vi "reward_behavior_michelle_visjitter_conswin_enticefx.vi"() -> ()   [LabVIEW 2019]
doc: "The myRIO Project template acquires acceleration data from the onboard accelerometer and displays the changes of acceleration values in a waveform chart."
uses:
  <vilib>/myRIO/Common/Instrument Driver Framework/Utilities/typedefs/Generic FPGA Reference.ctl
  <vilib>/myRIO/Common/Instrument Driver Framework/Utilities/typedefs/myRIO v1.0 Reference.ctl
  <vilib>/myRIO/Common/Instrument Driver Framework/Utilities/typedefs/Hardware Version Enum.ctl
  <vilib>/myRIO/Common/Instrument Driver Framework/Utilities/typedefs/myRIO Generic Hardware Reference.ctl
  <vilib>/userdefined/High Color/nirio_resource_hc.ctl
  <vilib>/myRIO/Common/Instrument Driver Framework/Utilities/vis/Is FPGA Ref Available.vi
  <vilib>/myRIO/Common/Instrument Driver Framework/myRIO v1.0/Encoder/typedefs/Encoder Signal Mode.ctl
  <vilib>/myRIO/Common/Instrument Driver Framework/myRIO v1.0/Encoder/typedefs/Encoder Channels Enum.ctl
  <vilib>/myRIO/Instrument Drivers/Onboard IO/Encoder/typedefs/Encoder Reference.ctl
  <vilib>/myRIO/Instrument Drivers/Onboard IO/Encoder/Encoder.lvlib
  <vilib>/myRIO/Instrument Drivers/Onboard IO/Encoder/vis/Read.vi
  <vilib>/myRIO/Common/Instrument Driver Framework/myRIO v1.0/Encoder/typedefs/Encoder Configuration v1.0.ctl
  <vilib>/myRIO/Common/Instrument Driver Framework/myRIO v1.0/Encoder/vis/myRIO v1.1 Open Encoder.vi
  <vilib>/myRIO/Common/Instrument Driver Framework/myRIO v1.0/Encoder/vis/myRIO v1.0 Configure Encoder.vi
  <vilib>/myRIO/Instrument Drivers/Onboard IO/Encoder/vis/myRIO Encoder Open.xnode
  <vilib>/myRIO/Express VI/Onboard IO/Encoder/Encoder Express VI.xnode
  <vilib>/myRIO/Express VI/Onboard IO/DI/DI Express VI.xnode
  <vilib>/myRIO/Instrument Drivers/Onboard IO/DIO/vis/Read.vi
  <vilib>/myRIO/Instrument Drivers/Onboard IO/DIO/DIO.lvlib
  <vilib>/myRIO/Common/Instrument Driver Framework/myRIO v1.0/DIO/typedefs/DIO Channels Enum.ctl
  <vilib>/myRIO/Common/Instrument Driver Framework/myRIO v1.0/DIO/typedefs/DIO Channels List.ctl
  <vilib>/myRIO/Instrument Drivers/Onboard IO/DIO/typedefs/DIO Reference.ctl
  <vilib>/myRIO/Instrument Drivers/Onboard IO/DIO/vis/myRIO DIO Open.xnode
  <vilib>/myRIO/Common/Instrument Driver Framework/myRIO v1.0/DIO/vis/myRIO v1.1 Open DIO.vi
  <vilib>/myRIO/Instrument Drivers/Onboard IO/DIO/vis/Write.vi
  <vilib>/myRIO/Express VI/Onboard IO/DO/DO Express VI.xnode
  <vilib>/Analysis/Matrix/Datatypes/RealMatrix.ctl
  <vilib>/Analysis/Matrix/NI_Matrix.lvlib
panel:
  out "ContrastChoice":dbl
  out "Enticements":i32
  in  "Entice":bool
  out "Misses":i32
  out "GoAhead":bool
  out "TimeOutDuration":i32
  out "ActiveTime":dbl
  out "ConsumptionGo":bool=TRUE
  out "Consumption_Period":i32
  out "Watch_Display":bool=TRUE
  in  "Give reward":bool
  out "Timings":dbl[](array[numeric])
  out "ISI":dbl
  out "ISI start time":dbl
  out "Time_out":bool=TRUE
  out "Time since lick":dbl
  out "Time of last lick":dbl
  out "Rewarded trials":dbl[](array[numeric])
  out "Rewards":u16
  out "Active Trial":bool
  out "Array temp2":T1
  out "Stimuli Loaded":bool
  out "Stim_ID":dbl[](array[numeric])
  out "Reward_mat":dbl[](array[numeric])
  out "Reward":bool=TRUE
  out "Frame clock":i32
  out "Licks":u32
  out "Lick":bool
  out "Time":dbl
  out "Stop":bool
  in  "Frames to collect":u32
  out "Overflow?":bool
  out "Counter Value":i32
  out "Velocity":dbl
  out "Velocity Plot":dbl[](graph)
  out "Velocity array":dbl[](array[numeric])
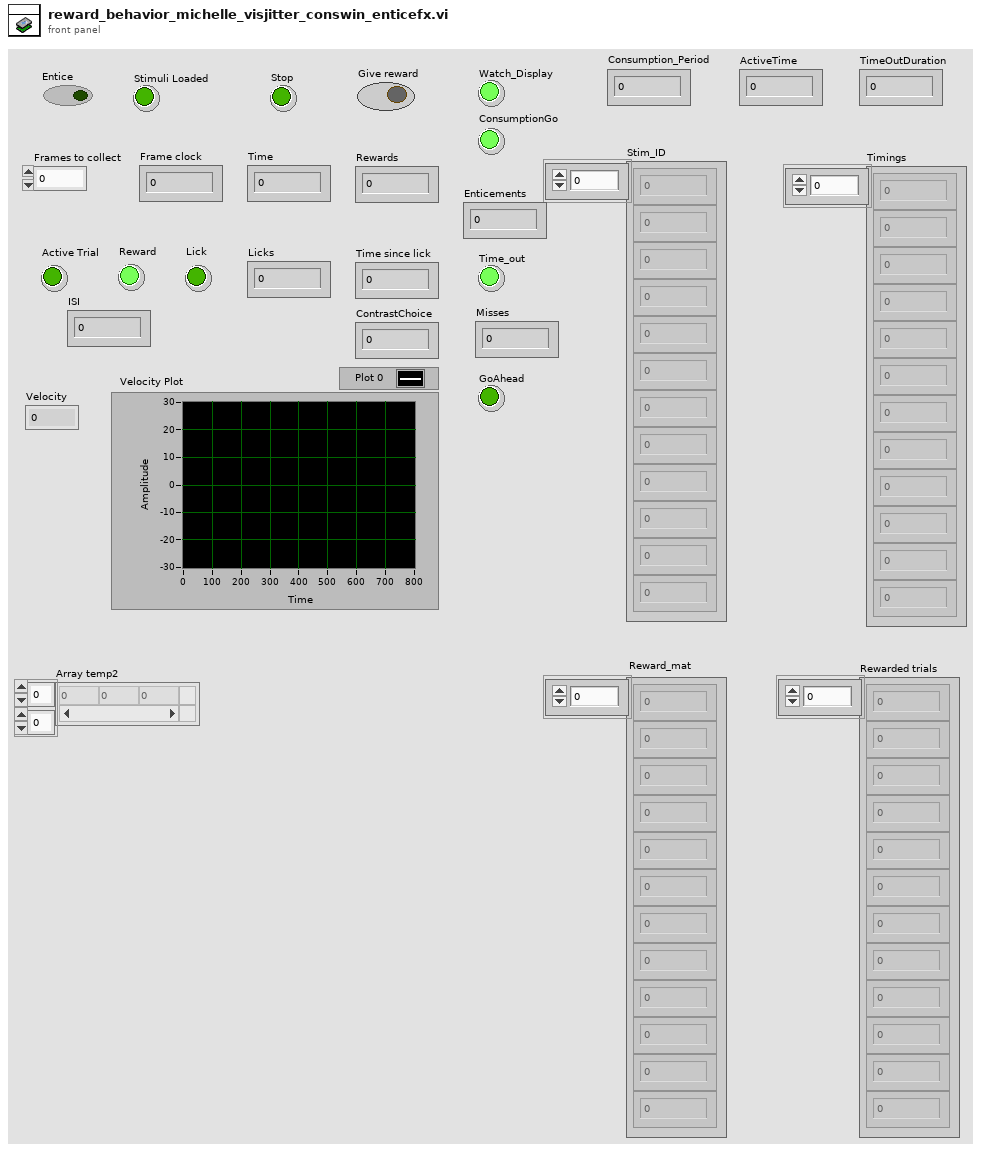
[diagram p1: front panel]
types:
  T1 = typedef "NI_Matrix.lvlib/RealMatrix.ctl" = dbl[][]
  T2 = typedef "Encoder.lvlib/Encoder Reference.ctl" = cluster{"myRIO Reference":T3, "Encoder Channels Enum":T7}
  T3 = typedef "myRIO Generic Hardware Reference.ctl" = cluster{"myRIO Model":T4, "myRIO Hardware Reference":T5}
  T4 = typedef "Hardware Version Enum.ctl" = enum16{"Unknown", "myRIO-1900", "myRIO-1950", "roboRIO", "NI ELVIS RIO CM", "ELVIS III"}
  T5 = typedef "myRIO v1.0 Reference.ctl" = cluster{"Generic FPGA Reference":T6, "Allow multiple opens":bool}
  T6 = typedef "Generic FPGA Reference.ctl" = refnum<k20>
  T7 = typedef "Encoder Channels Enum.ctl" = enum16{"Not Connected", "C/ENC0", "C/ENC1", "A/ENC", "A/ENC0", "A/ENC1", "A/ENC2", "A/ENC3", "A/ENC4", "A/ENC5", "A/ENC6", "A/ENC7", "A/ENC8", "A/ENC9", "B/ENC", "B/ENC0", "B/ENC1", "B/ENC2", "B/ENC3", "B/ENC4", "B/ENC5", "B/ENC6", "B/ENC7", "B/ENC8", "B/ENC9", "DIO/ENC0", "DIO/ENC1", "DIO/ENC2", "DIO/ENC3", "DIO/ENC4"}
  T8 = typedef "Encoder Signal Mode.ctl" = enum16{"Quadrature phase signal", "Step and direction signal"}
  T9 = typedef "nirio_resource_hc.ctl" = tag
  T10 = typedef "DIO.lvlib/DIO Reference.ctl" = cluster{"myRIO Reference":T3, "DIO Channels List":T11}
  T11 = typedef "DIO Channels List.ctl" = T12[]
  T12 = typedef "DIO Channels Enum.ctl" = enum16{"Not Connected", "C/DIO0", "C/DIO1", "C/DIO2", "C/DIO3", "C/DIO4", "C/DIO5", "C/DIO6", "C/DIO7", "A/DIO0", "A/DIO1", "A/DIO2", "A/DIO3", "A/DIO4", "A/DIO5", "A/DIO6", "A/DIO7", "A/DIO8", "A/DIO9", "A/DIO10", "A/DIO11", "A/DIO12", "A/DIO13", "A/DIO14", "A/DIO15", "A/DIO16", "A/DIO17", "A/DIO18", "A/DIO19", "B/DIO0", "B/DIO1", "B/DIO2", "B/DIO3", "B/DIO4", "B/DIO5", "B/DIO6", "B/DIO7", "B/DIO8", "B/DIO9", "B/DIO10", "B/DIO11", "B/DIO12", "B/DIO13", "B/DIO14", "B/DIO15", "B/DIO16", "B/DIO17", "B/DIO18", "B/DIO19", "LED0", "LED1", "LED2", "LED3", "Button0", "DIO/DIO0", "DIO/DIO1", "DIO/DIO2", "DIO/DIO3", "DIO/DIO4", "DIO/DIO5", "DIO/DIO6", "DIO/DIO7", "DIO/DIO8", "DIO/DIO9", "SPI/CS0", "SPI/CS1", "SPI/CS2", "SPI/CS3", "LED RADIO (Green)", "LED RADIO (Red)", "LED COMM (Green)", "LED COMM (Red)", "LED MODE (Green)", "LED MODE (Red)"}
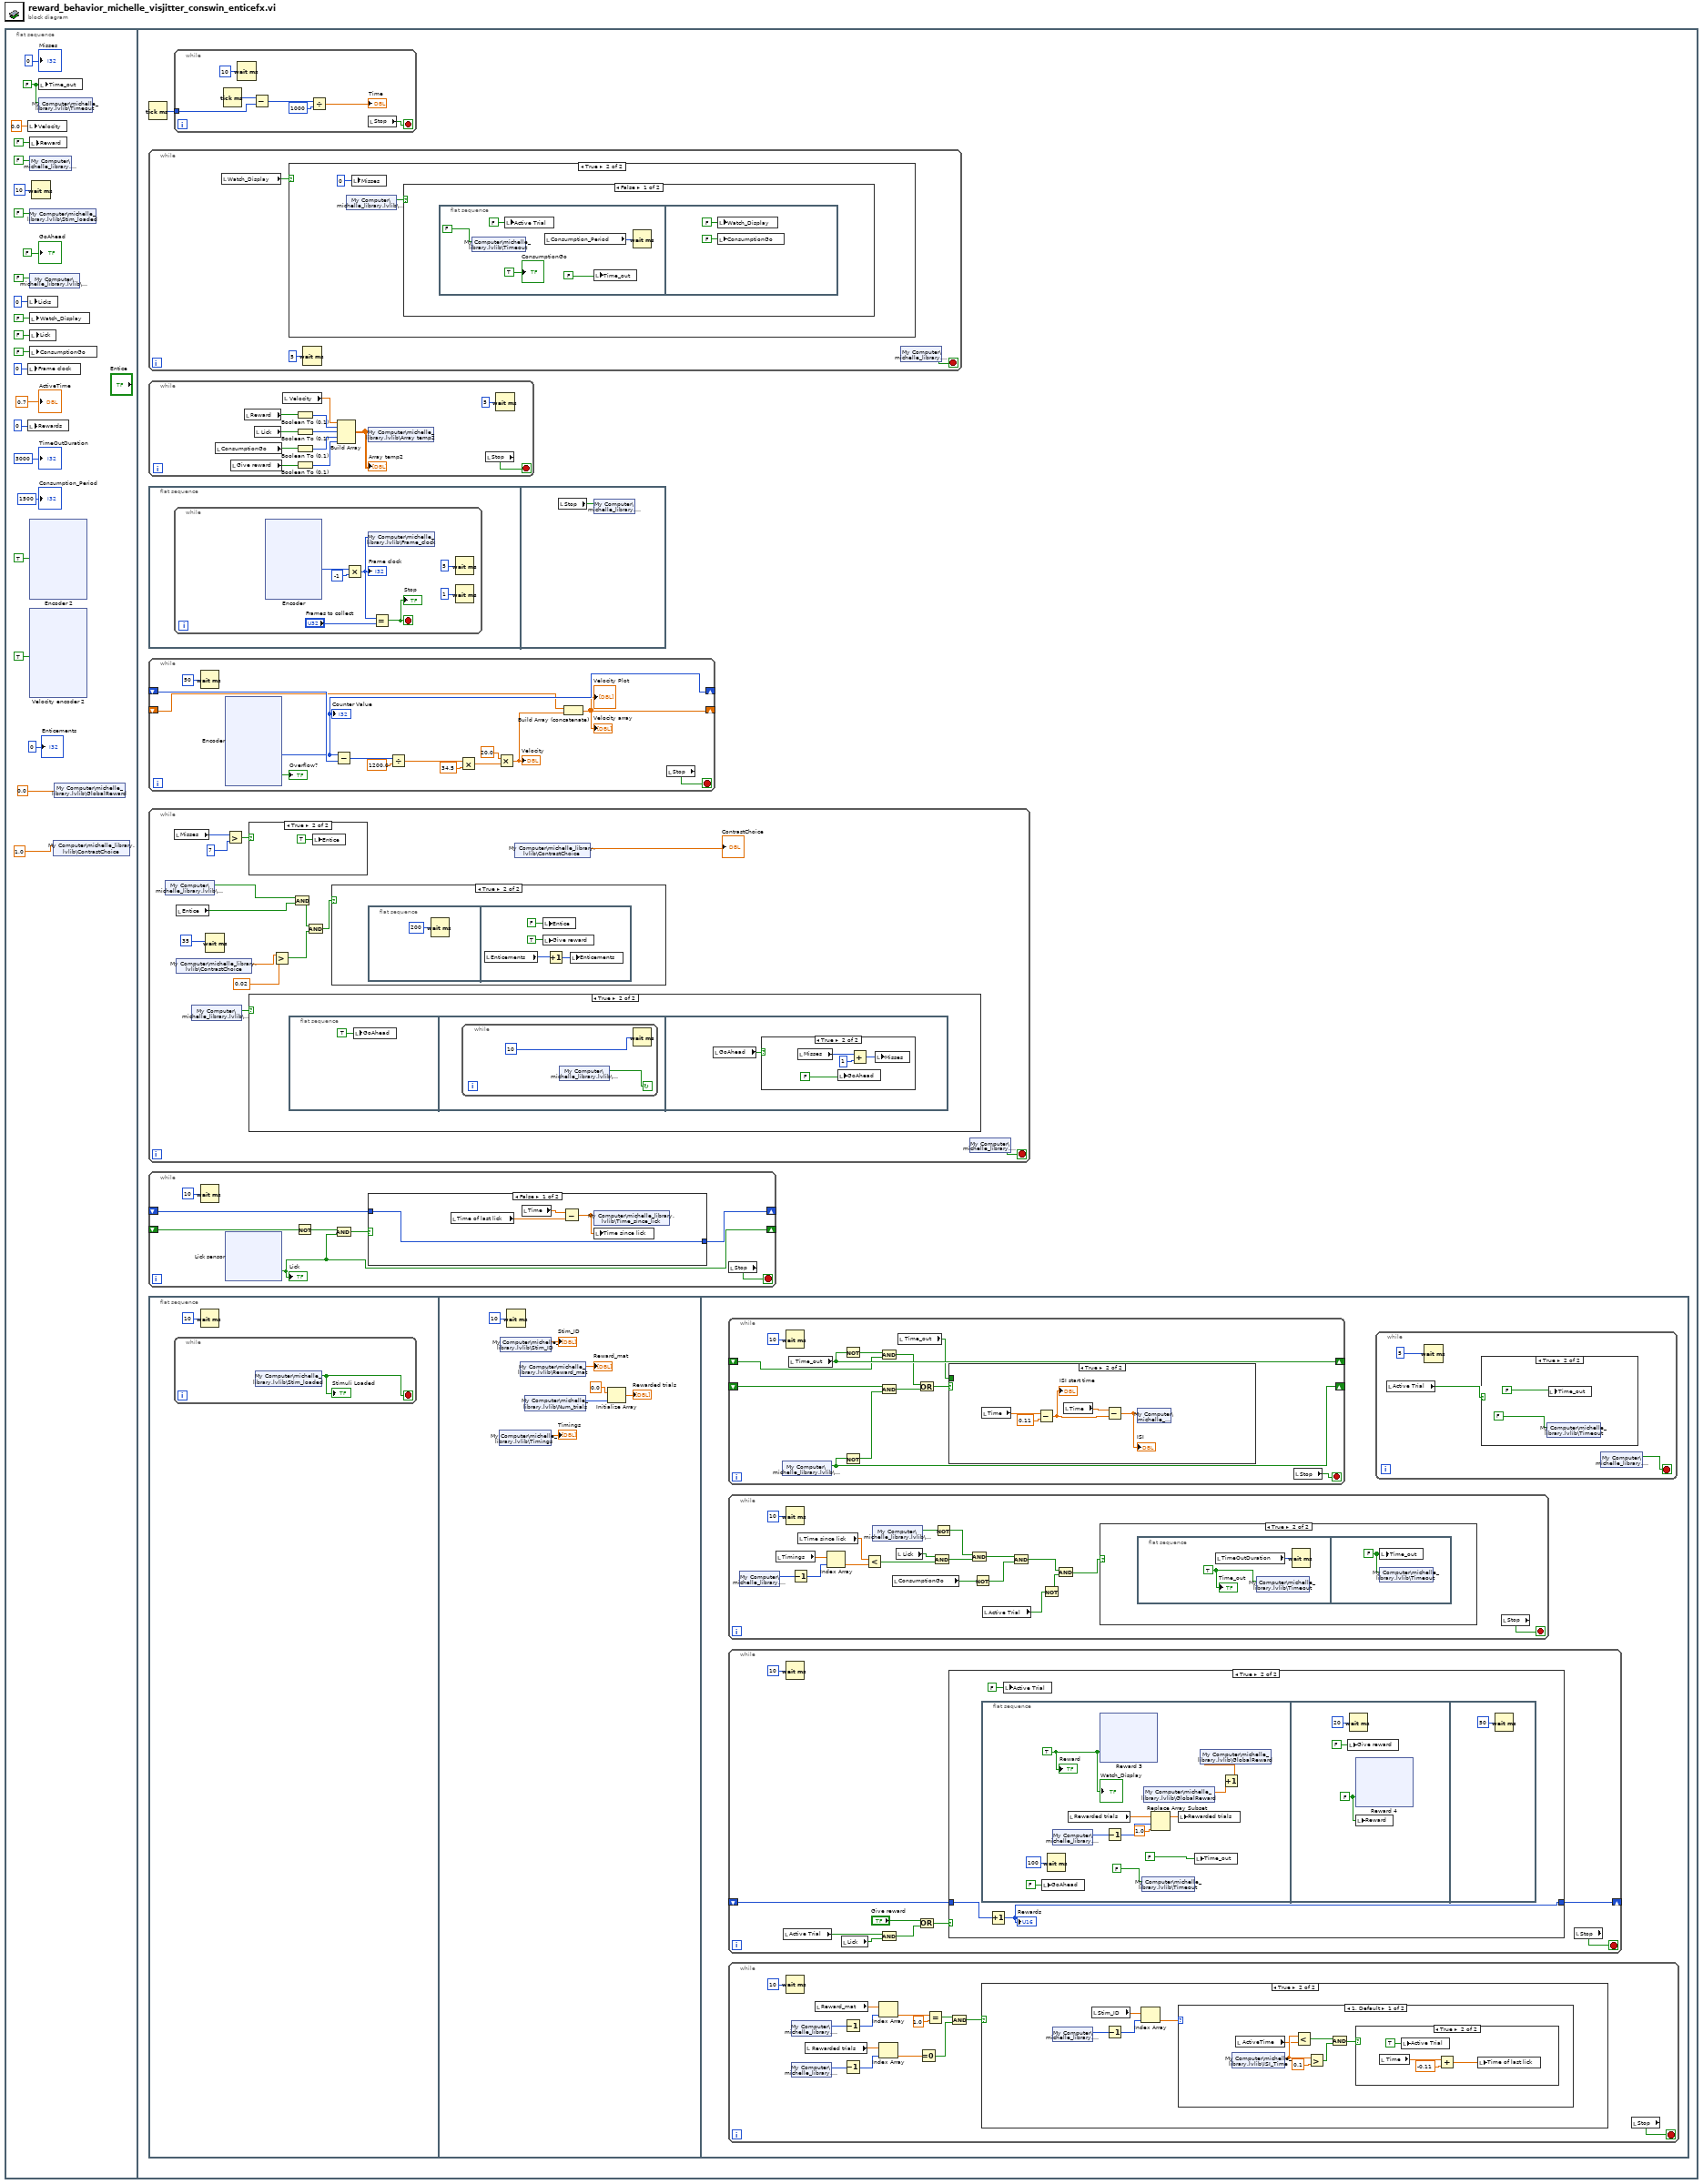
[diagram p0: block diagram]
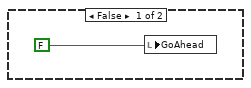
[diagram p4: hidden frame]
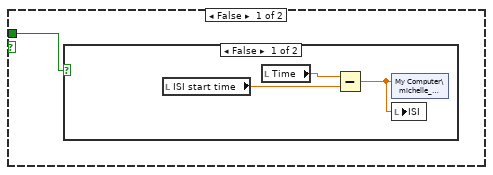
[diagram p10: hidden frame]
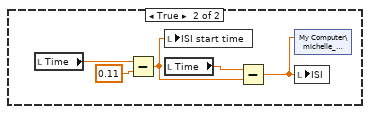
[diagram p11: hidden frame]
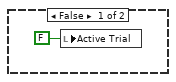
[diagram p12: hidden frame]
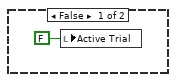
[diagram p13: hidden frame]
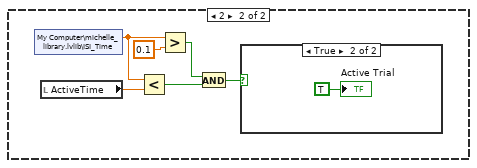
[diagram p14: hidden frame]
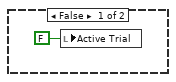
[diagram p15: hidden frame]
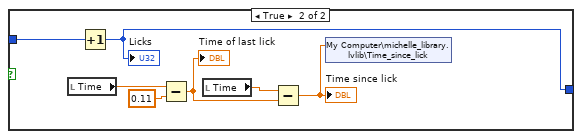
[diagram p17: hidden frame]
diagram:
  n1 = flat-sequence {
    frame #0 {
      w11 = FALSE ("Time_out")
      n2 = local write "Velocity"(0.0 ("Velocity")) -> ()
      n3 = local write "Licks"(u32 0 ("Licks")) -> ()
      n4 = local write "Frame clock"(u32 0 ("Frames")) -> ()
      n5 = local write "Rewards"(u16 0 ("Rewards")) -> ()
      n6 = local write "Reward"(FALSE ("Give reward")) -> ()
      n7 = shared-variable "My Computer\\michelle_library.lvlib\\Stop"(FALSE ("Stop")) -> ()  [unwired: 1 in, 1 out]
      n8 = shared-variable "My Computer\\michelle_library.lvlib\\Stim_loaded"(FALSE ("Stim_loaded")) -> ()  [unwired: 1 in, 1 out]
      n9 = shared-variable "My Computer\\michelle_library.lvlib\\Display"(FALSE ("Display")) -> ()  [unwired: 1 in, 1 out]
      n10 = local write "Watch_Display"(FALSE ("Watch_Display")) -> ()
      n11 = local write "Lick"(FALSE ("Lick")) -> ()
      n12 = local write "ConsumptionGo"(FALSE ("ConsumptionGo")) -> ()
      n13 = xnode "Encoder 2"("Reset Counter"=TRUE) -> ()  [unwired: 1 in, 4 out]
      n14 = xnode "Velocity encoder 2"("Reset Counter"=TRUE) -> ()  [unwired: 1 in, 4 out]
      n15 = Wait (ms)(milliseconds to wait=u32 10) -> ()  [unwired: 1 out]
      n16 = local write "Time_out"(w11) -> ()
      n17 = shared-variable "My Computer\\michelle_library.lvlib\\Timeout"(w11) -> ()  [unwired: 1 in, 1 out]
      n18 = shared-variable "My Computer\\michelle_library.lvlib\\ContrastChoice"(1.0) -> ()  [unwired: 1 in, 1 out]
      n19 = shared-variable "My Computer\\michelle_library.lvlib\\GlobalReward"(0.0) -> ()  [unwired: 1 in, 1 out]
      "Consumption_Period" <- 1500
      "ActiveTime" <- 0.7
      "TimeOutDuration" <- 3000
      "GoAhead" <- FALSE
      "Misses" <- 0
      "Enticements" <- 0
    }
    frame #1 {
      n20 = Tick Count (ms)() -> (millisecond timer value=w116:u32)
      n21 = while {
        stop <- w148 stop-if-true
        n22 = local read "Watch_Display"() -> (w147:bool)
        n23 = case shown="True" w147 {
          frame False {
          }
          frame True {
            n24 = shared-variable "My Computer\\michelle_library.lvlib\\Display"() -> (w150:bool)  [unwired: 1 in, 1 out]
            n25 = local write "Misses"(0) -> ()
            n26 = case shown="False" w150 {
              frame False {
                n27 = flat-sequence {
                  frame #0 {
                    n28 = shared-variable "My Computer\\michelle_library.lvlib\\Timeout"(FALSE) -> ()  [unwired: 1 in, 1 out]
                    n29 = local write "Active Trial"(FALSE) -> ()
                    n30 = local read "Consumption_Period"() -> (w155:i32)
                    n31 = local write "Time_out"(FALSE) -> ()
                    n32 = Wait (ms)(milliseconds to wait=w155) -> ()  [unwired: 1 out]
                    "ConsumptionGo" <- TRUE
                  }
                  frame #1 {
                    n33 = local write "Watch_Display"(FALSE ("Watch_Display")) -> ()
                    n34 = local write "ConsumptionGo"(FALSE ("ConsumptionGo")) -> ()
                  }
                }
              }
              frame True {
              }
            }
          }
        }
        n35 = Wait (ms)(milliseconds to wait=u32 5) -> ()  [unwired: 1 out]
        n36 = shared-variable "My Computer\\michelle_library.lvlib\\Stop"() -> (w148:bool)  [unwired: 1 in, 1 out]
      }
      n37 = while {
        stop <- w163 stop-if-true
        n38 = local read "ConsumptionGo"() -> (w161:bool)
        n39 = local read "Give reward"() -> (w160:bool)
        n40 = local read "Reward"() -> (w168:bool)
        n41 = local read "Lick"() -> (w169:bool)
        n42 = local read "Velocity"() -> (w167:dbl)
        n43 = Boolean To (0,1)(Boolean=w168) -> (0, 1=w166:i16)
        n44 = Boolean To (0,1)(Boolean=w169) -> (0, 1=w165:i16)
        n45 = Boolean To (0,1)(Boolean=w161) -> (0, 1=w159:i16)
        n46 = Boolean To (0,1)(Boolean=w160) -> (0, 1=w158:i16)
        n47 = Build Array(w167, w166, w165, w159, w158) -> (w162:T1)
        "Array temp2" <- w162
        n48 = shared-variable "My Computer\\michelle_library.lvlib\\Array temp2"(w162) -> ()  [unwired: 1 in, 1 out]
        n49 = local read "Stop"() -> (w163:bool)
        n50 = Wait (ms)(milliseconds to wait=u32 5) -> ()  [unwired: 1 out]
      }
      n51 = flat-sequence {
        frame #0 {
          n52 = while {
            stop <- w370 stop-if-true
            n53 = xnode "Encoder"() -> ("Counter Value"=w374:i32)  [unwired: 2 in, 3 out]
            n54 = Multiply(x=w374, y=-1) -> (x*y=w369:i32)
            "Frame clock" <- w369
            n55 = shared-variable "My Computer\\michelle_library.lvlib\\Frame_clock"(w369) -> ()  [unwired: 1 in, 1 out]
            n56 = Equal?(x=w369, y="Frames to collect") -> (x = y?=w370:bool)
            "Stop" <- w370
            n57 = Wait (ms)(milliseconds to wait=u32 5) -> ()  [unwired: 1 out]
            n58 = Wait (ms)(milliseconds to wait=u32 1) -> ()  [unwired: 1 out]
          }
        }
        frame #1 {
          n59 = local read "Stop"() -> (w422:bool)
          n60 = shared-variable "My Computer\\michelle_library.lvlib\\Stop"(w422) -> ()  [unwired: 1 in, 1 out]
        }
      }
      n61 = while {
        shift-right: [w487] -> _
        shift-left: _ -> [w488]
        shift-right: [w479] -> _
        shift-left: _ -> [w478]
        stop <- w477 stop-if-true
        n62 = Wait (ms)(milliseconds to wait=u32 50) -> ()  [unwired: 1 out]
        n63 = xnode "Encoder"() -> ("Counter Value"=w487:i32, "Overflow?"=→"Overflow?":bool)  [unwired: 2 in, 2 out]
        "Counter Value" <- w487
        n64 = Subtract(x=w487, y=w488) -> (x-y=w480:i32)
        n65 = Divide(x=w480, y=1200.0 ("600")) -> (x/y=w485:dbl)
        n66 = Multiply(x=w485, y=34.5) -> (x*y=w483:dbl)
        n67 = Multiply(x=20.0, y=w483) -> (x*y=w481:dbl)
        "Velocity" <- w481
        n68 = Build Array (concatenate)(w478, w481) -> (w479:dbl[])
        "Velocity Plot" <- w479
        "Velocity array" <- w479
        n69 = local read "Stop"() -> (w477:bool)
      }
      n70 = while {
        stop <- w130 stop-if-true
        n71 = shared-variable "My Computer\\michelle_library.lvlib\\Display"() -> (w125:bool)  [unwired: 1 in, 1 out]
        n72 = local read "Misses"() -> (w128:i32)
        n73 = shared-variable "My Computer\\michelle_library.lvlib\\ContrastChoice"() -> (w122:dbl)  [unwired: 1 in, 1 out]
        n74 = local read "Entice"() -> (w124:bool)
        n75 = shared-variable "My Computer\\michelle_library.lvlib\\Display"() -> (w129:bool)  [unwired: 1 in, 1 out]
        n76 = Wait (ms)(milliseconds to wait=35) -> ()  [unwired: 1 out]
        n77 = Greater?(x=w128, y=7) -> (0:w126:bool)
        n78 = case shown="True" w126 {
          frame False {
          }
          frame True {
            n79 = local write "Entice"(TRUE) -> ()
          }
        }
        n80 = case shown="True" w129 {
          frame False {
            n81 = local write "GoAhead"(FALSE) -> ()
          }
          frame True {
            n82 = flat-sequence {
              frame #0 {
                n83 = local write "GoAhead"(TRUE) -> ()
              }
              frame #1 {
                n84 = while {
                  stop <- w140 continue-if-true
                  n85 = shared-variable "My Computer\\michelle_library.lvlib\\Display"() -> (w140:bool)  [unwired: 1 in, 1 out]
                  n86 = Wait (ms)(milliseconds to wait=10) -> ()  [unwired: 1 out]
                }
              }
              frame #2 {
                n87 = local read "GoAhead"() -> (w141:bool)
                n88 = case shown="True" w141 {
                  frame False {
                  }
                  frame True {
                    n89 = local read "Misses"() -> (w145:i32)
                    n90 = local write "GoAhead"(FALSE) -> ()
                    n91 = Add(x=w145, y=1) -> (x+y=w143:i32)
                    n92 = local write "Misses"(w143) -> ()
                  }
                }
              }
            }
          }
        }
        n93 = Greater?(x=w122, y=0.02) -> (0:w119:bool)
        n94 = And(x=w125, y=w124) -> (x .and. y?=w120:bool)
        n95 = And(x=w120, y=w119) -> (x .and. y?=w118:bool)
        n96 = case shown="True" w118 {
          frame False {
          }
          frame True {
            n97 = flat-sequence {
              frame #0 {
                n98 = Wait (ms)(milliseconds to wait=200) -> ()  [unwired: 1 out]
              }
              frame #1 {
                n99 = local read "Enticements"() -> (w133:i32)
                n100 = local write "Entice"(FALSE) -> ()
                n101 = local write "Give reward"(TRUE) -> ()
                n102 = Increment(x=w133) -> (x+1=w132:i32)
                n103 = local write "Enticements"(w132) -> ()
              }
            }
          }
        }
        n104 = shared-variable "My Computer\\michelle_library.lvlib\\ContrastChoice"() -> (→"ContrastChoice":dbl)  [unwired: 1 in, 1 out]
        n105 = shared-variable "My Computer\\michelle_library.lvlib\\Stop"() -> (w130:bool)  [unwired: 1 in, 1 out]
      }
      n106 = while {
        shift-right: [w429] -> _
        shift-left: _ -> [w428]
        shift-right: [w423] -> _
        shift-left: _ -> [w426]
        stop <- w427 stop-if-true
        n107 = Wait (ms)(milliseconds to wait=u32 10) -> ()  [unwired: 1 out]
        n108 = xnode "Lick sensor"() -> ("C/DIO1 (DIO1)"=w423:bool)  [unwired: 1 in, 1 out]
        "Lick" <- w423
        n109 = Not(x=w426) -> (.not. x?=w425:bool)
        n110 = And(x=w425, y=w423) -> (x .and. y?=w424:bool)
        n111 = case shown="False" w424 {
          tunnel: [w434 w441] -> w429
          tunnel: w428 -> [w434 w440]
          frame False {
            n112 = local read "Time of last lick"() -> (w432:dbl)
            n113 = local read "Time"() -> (w433:dbl)
            n114 = Subtract(x=w433, y=w432) -> (x-y=w431:dbl)
            n115 = shared-variable "My Computer\\michelle_library.lvlib\\Time_since_lick"(w431) -> ()  [unwired: 1 in, 1 out]
            n116 = local write "Time since lick"(w431) -> ()
          }
          frame True {
            n117 = local read "Time"() -> (w437:dbl)
            n118 = Increment(x=w440) -> (x+1=w441:u32)
            "Licks" <- w441
            n119 = Subtract(x=w437, y=0.11) -> (x-y=w435:dbl)
            "Time of last lick" <- w435
            n120 = local read "Time"() -> (w439:dbl)
            n121 = Subtract(x=w439, y=w435) -> (x-y=w438:dbl)
            "Time since lick" <- w438
            n122 = shared-variable "My Computer\\michelle_library.lvlib\\Time_since_lick"(w438) -> ()  [unwired: 1 in, 1 out]
          }
        }
        n123 = local read "Stop"() -> (w427:bool)
      }
      n124 = flat-sequence {
        frame #0 {
          n125 = while {
            stop <- w171 stop-if-true
            n126 = shared-variable "My Computer\\michelle_library.lvlib\\Stim_loaded"() -> (w171:bool)  [unwired: 1 in, 1 out]
            "Stimuli Loaded" <- w171
          }
          n127 = Wait (ms)(milliseconds to wait=u32 10) -> ()  [unwired: 1 out]
        }
        frame #1 {
          n128 = shared-variable "My Computer\\michelle_library.lvlib\\Timings"() -> (→"Timings":dbl[])  [unwired: 1 in, 1 out]
          n129 = shared-variable "My Computer\\michelle_library.lvlib\\Stim_ID"() -> (→"Stim_ID":dbl[])  [unwired: 1 in, 1 out]
          n130 = Wait (ms)(milliseconds to wait=u32 10) -> ()  [unwired: 1 out]
          n131 = shared-variable "My Computer\\michelle_library.lvlib\\Reward_mat"() -> (→"Reward_mat":dbl[])  [unwired: 1 in, 1 out]
          n132 = shared-variable "My Computer\\michelle_library.lvlib\\Num_trials"() -> (w175:u32)  [unwired: 1 in, 1 out]
          n133 = Initialize Array(0.0 ("element"), w175) -> (→"Rewarded trials":dbl[])
        }
        frame #2 {
          n134 = while {
            shift-right: [w216] -> _
            shift-left: _ -> [w214]
            shift-right: [w212] -> _
            shift-left: _ -> [w211]
            stop <- w217 stop-if-true
            n135 = shared-variable "My Computer\\michelle_library.lvlib\\Display"() -> (w212:bool)  [unwired: 1 in, 1 out]
            n136 = Wait (ms)(milliseconds to wait=u32 10) -> ()  [unwired: 1 out]
            n137 = local read "Time_out"() -> (w216:bool)
            n138 = Not(x=w216) -> (.not. x?=w215:bool)
            n139 = Not(x=w212) -> (.not. x?=w210:bool)
            n140 = And(x=w215, y=w214) -> (x .and. y?=w209:bool)
            n141 = And(x=w211, y=w210) -> (x .and. y?=w208:bool)
            n142 = local read "Time_out"() -> (w213:bool)
            n143 = Or(x=w209, y=w208) -> (x .or. y?=w207:bool)
            n144 = case shown="True" w207 {
              tunnel: w213 -> [w218 _]
              frame False {
                n145 = case shown="False" w218 {
                  frame False {
                    n146 = local read "ISI start time"() -> (w221:dbl)
                    n147 = local read "Time"() -> (w220:dbl)
                    n148 = Subtract(x=w220, y=w221) -> (x-y=w219:dbl)
                    n149 = shared-variable "My Computer\\michelle_library.lvlib\\ISI"(w219) -> ()  [unwired: 1 in, 1 out]
                    n150 = local write "ISI"(w219) -> ()
                  }
                  frame True {
                    n151 = local read "Time"() -> (w226:dbl)
                    n152 = Subtract(x=w226, y=0.11) -> (x-y=w223:dbl)
                    n153 = local write "ISI start time"(w223) -> ()
                    n154 = local read "Time"() -> (w224:dbl)
                    n155 = Subtract(x=w224, y=w223) -> (x-y=w222:dbl)
                    n156 = shared-variable "My Computer\\michelle_library.lvlib\\ISI"(w222) -> ()  [unwired: 1 in, 1 out]
                    n157 = local write "ISI"(w222) -> ()
                  }
                }
              }
              frame True {
                n158 = local read "Time"() -> (w231:dbl)
                n159 = Subtract(x=w231, y=0.11) -> (x-y=w228:dbl)
                "ISI start time" <- w228
                n160 = local read "Time"() -> (w229:dbl)
                n161 = Subtract(x=w229, y=w228) -> (x-y=w227:dbl)
                "ISI" <- w227
                n162 = shared-variable "My Computer\\michelle_library.lvlib\\ISI"(w227) -> ()  [unwired: 1 in, 1 out]
              }
            }
            n163 = local read "Stop"() -> (w217:bool)
          }
          n164 = while {
            stop <- w202 stop-if-true
            n165 = shared-variable "My Computer\\michelle_library.lvlib\\Trial"() -> (w192:u32)  [unwired: 1 in, 1 out]
            n166 = local read "Timings"() -> (w194:dbl[])
            n167 = Wait (ms)(milliseconds to wait=u32 10) -> ()  [unwired: 1 out]
            n168 = Decrement(x=w192) -> (x-1=w191:u32)
            n169 = local read "Time since lick"() -> (w201:dbl)
            n170 = Index Array(array=w194, index=w191) -> (element=w193:dbl)
            n171 = Less?(x=w201, y=w193) -> (x < y?=w200:bool)
            n172 = shared-variable "My Computer\\michelle_library.lvlib\\Display"() -> (w197:bool)  [unwired: 1 in, 1 out]
            n173 = local read "ConsumptionGo"() -> (w189:bool)
            n174 = local read "Lick"() -> (w199:bool)
            n175 = And(x=w199, y=w200) -> (x .and. y?=w195:bool)
            n176 = Not(x=w197) -> (.not. x?=w196:bool)
            n177 = And(x=w196, y=w195) -> (x .and. y?=w188:bool)
            n178 = Not(x=w189) -> (.not. x?=w190:bool)
            n179 = local read "Active Trial"() -> (w184:bool)
            n180 = And(x=w188, y=w190) -> (x .and. y?=w186:bool)
            n181 = Not(x=w184) -> (.not. x?=w187:bool)
            n182 = And(x=w186, y=w187) -> (x .and. y?=w185:bool)
            n183 = case shown="True" w185 {
              frame False {
              }
              frame True {
                n184 = flat-sequence {
                  frame #0 {
                    w204 = TRUE
                    n185 = local read "TimeOutDuration"() -> (w203:i32)
                    n186 = shared-variable "My Computer\\michelle_library.lvlib\\Timeout"(w204) -> ()  [unwired: 1 in, 1 out]
                    n187 = Wait (ms)(milliseconds to wait=w203) -> ()  [unwired: 1 out]
                    "Time_out" <- w204
                  }
                  frame #1 {
                    w205 = FALSE ("Timeout")
                    n188 = local write "Time_out"(w205) -> ()
                    n189 = shared-variable "My Computer\\michelle_library.lvlib\\Timeout"(w205) -> ()  [unwired: 1 in, 1 out]
                  }
                }
              }
            }
            n190 = local read "Stop"() -> (w202:bool)
          }
          n191 = while {
            shift-right: [w276] -> _
            shift-left: _ -> [w275]
            stop <- w278 stop-if-true
            n192 = local read "Active Trial"() -> (w273:bool)
            n193 = Wait (ms)(milliseconds to wait=u32 10) -> ()  [unwired: 1 out]
            n194 = local read "Lick"() -> (w274:bool)
            n195 = And(x=w273, y=w274) -> (x .and. y?=w272:bool)
            n196 = Or(x="Give reward", y=w272) -> (x .or. y?=w271:bool)
            n197 = case shown="True" w271 {
              tunnel: [w279 w282] -> w276
              tunnel: w275 -> [w279 w281]
              frame False {
              }
              frame True {
                n198 = flat-sequence {
                  frame #0 {
                    w293 = TRUE ("C/DIO0 (DIO0)")
                    n199 = local write "GoAhead"(FALSE) -> ()
                    n200 = Wait (ms)(milliseconds to wait=u32 100) -> ()  [unwired: 1 out]
                    n201 = shared-variable "My Computer\\michelle_library.lvlib\\Trial"() -> (w292:u32)  [unwired: 1 in, 1 out]
                    n202 = local read "Rewarded trials"() -> (w290:dbl[])
                    n203 = xnode "Reward 3"("C/DIO0 (DIO0)"=w293) -> ()  [unwired: 1 in, 1 out]
                    n204 = Decrement(x=w292) -> (x-1=w291:u32)
                    n205 = shared-variable "My Computer\\michelle_library.lvlib\\Timeout"(FALSE) -> ()  [unwired: 1 in, 1 out]
                    n206 = shared-variable "My Computer\\michelle_library.lvlib\\GlobalReward"() -> (w284:dbl)  [unwired: 1 in, 1 out]
                    n207 = Replace Array Subset(array=w290, new element=1.0 ("new element/subarray"), index=w291) -> (w288:dbl[])
                    n208 = local write "Rewarded trials"(w288) -> ()
                    n209 = local write "Time_out"(FALSE) -> ()
                    n210 = Increment(x=w284) -> (x+1=w283:dbl)
                    n211 = shared-variable "My Computer\\michelle_library.lvlib\\GlobalReward"(w283) -> ()  [unwired: 1 in, 1 out]
                    "Reward" <- w293
                    "Watch_Display" <- w293
                  }
                  frame #1 {
                    w332 = FALSE ("C/DIO0 (DIO0)")
                    n212 = local write "Give reward"(FALSE ("Give reward")) -> ()
                    n213 = Wait (ms)(milliseconds to wait=u32 20) -> ()  [unwired: 1 out]
                    n214 = xnode "Reward 4"("C/DIO0 (DIO0)"=w332) -> ()  [unwired: 1 in, 1 out]
                    n215 = local write "Reward"(w332) -> ()
                  }
                  frame #2 {
                    n216 = Wait (ms)(milliseconds to wait=u32 50) -> ()  [unwired: 1 out]
                  }
                }
                n217 = Increment(x=w281) -> (x+1=w282:u16)
                "Rewards" <- w282
                n218 = local write "Active Trial"(FALSE ("Active Trial")) -> ()
              }
            }
            n219 = local read "Stop"() -> (w278:bool)
          }
          n220 = while {
            stop <- w245 stop-if-true
            n221 = Wait (ms)(milliseconds to wait=u32 10) -> ()  [unwired: 1 out]
            n222 = shared-variable "My Computer\\michelle_library.lvlib\\Trial"() -> (w241:u32)  [unwired: 1 in, 1 out]
            n223 = shared-variable "My Computer\\michelle_library.lvlib\\Trial"() -> (w237:u32)  [unwired: 1 in, 1 out]
            n224 = local read "Rewarded trials"() -> (w238:dbl[])
            n225 = local read "Reward_mat"() -> (w240:dbl[])
            n226 = Decrement(x=w241) -> (x-1=w242:u32)
            n227 = Decrement(x=w237) -> (x-1=w236:u32)
            n228 = Index Array(array=w240, index=w242) -> (element=w243:dbl)
            n229 = Index Array(array=w238, index=w236) -> (element=w235:dbl)
            n230 = Equal To 0?(x=w235) -> (x = 0?=w234:bool)
            n231 = Equal?(x=w243, y=1.0) -> (x = y?=w233:bool)
            n232 = And(x=w233, y=w234) -> (x .and. y?=w232:bool)
            n233 = case shown="True" w232 {
              frame False {
                n234 = local write "Active Trial"(FALSE ("Active_trial")) -> ()
              }
              frame True {
                n235 = shared-variable "My Computer\\michelle_library.lvlib\\Trial"() -> (w248:u32)  [unwired: 1 in, 1 out]
                n236 = local read "Stim_ID"() -> (w250:dbl[])
                n237 = Decrement(x=w248) -> (x-1=w249:u32)
                n238 = Index Array(array=w250, index=w249) -> (element=w247:dbl)
                n239 = case shown="1, Default" w247 {
                  frame 1, Default {
                    n240 = shared-variable "My Computer\\michelle_library.lvlib\\ISI_Time"() -> (w256:dbl)  [unwired: 1 in, 1 out]
                    n241 = local read "ActiveTime"() -> (w251:dbl)
                    n242 = Less?(x=w256, y=w251) -> (x < y?=w254:bool)
                    n243 = Greater?(x=w256, y=0.1) -> (0:w253:bool)
                    n244 = And(x=w254, y=w253) -> (x .and. y?=w252:bool)
                    n245 = case shown="True" w252 {
                      frame False {
                        n246 = local write "Active Trial"(FALSE ("Active Trial")) -> ()
                      }
                      frame True {
                        n247 = local read "Time"() -> (w260:dbl)
                        n248 = local write "Active Trial"(TRUE ("Active Trial")) -> ()
                        n249 = Add(x=w260, y=-0.11) -> (x+y=w258:dbl)
                        n250 = local write "Time of last lick"(w258) -> ()
                      }
                    }
                  }
                  frame 2 {
                    n251 = shared-variable "My Computer\\michelle_library.lvlib\\ISI_Time"() -> (w266:dbl)  [unwired: 1 in, 1 out]
                    n252 = local read "ActiveTime"() -> (w262:dbl)
                    n253 = Less?(x=w266, y=w262) -> (x < y?=w264:bool)
                    n254 = Greater?(x=w266, y=0.1) -> (0:w265:bool)
                    n255 = And(x=w265, y=w264) -> (x .and. y?=w263:bool)
                    n256 = case shown="True" w263 {
                      frame False {
                        n257 = local write "Active Trial"(FALSE ("Active Trial")) -> ()
                      }
                      frame True {
                        "Active Trial" <- TRUE ("Active Trial")
                      }
                    }
                  }
                }
              }
            }
            n258 = local read "Stop"() -> (w245:bool)
          }
          n259 = while {
            stop <- w181 stop-if-true
            n260 = local read "Active Trial"() -> (w180:bool)
            n261 = Wait (ms)(milliseconds to wait=5) -> ()  [unwired: 1 out]
            n262 = case shown="True" w180 {
              frame False {
              }
              frame True {
                n263 = shared-variable "My Computer\\michelle_library.lvlib\\Timeout"(FALSE) -> ()  [unwired: 1 in, 1 out]
                n264 = local write "Time_out"(FALSE) -> ()
              }
            }
            n265 = shared-variable "My Computer\\michelle_library.lvlib\\Stop"() -> (w181:bool)  [unwired: 1 in, 1 out]
          }
        }
      }
      n266 = while {
        tunnel: w116 -> [w542]
        stop <- w540 stop-if-true
        n267 = Tick Count (ms)() -> (millisecond timer value=w543:u32)
        n268 = Wait (ms)(milliseconds to wait=u32 10) -> ()  [unwired: 1 out]
        n269 = Subtract(x=w543, y=w542) -> (x-y=w539:u32)
        n270 = Divide(x=w539, y=u32 1000) -> (x/y=→"Time":dbl)
        n271 = local read "Stop"() -> (w540:bool)
      }
    }
  }
